vi "Initialize Source Channels.vi"(8 "error in (no error)":errorcluster, 10 "Source Channels":string[](array[string]), 11 "Session in":refnum<k15>) -> (0 "error out":errorcluster, 3 "Session out":refnum<k15>)   [LabVIEW 2020, in "NI-SWITCH Messaging.lvlib" / "NI-SWITCH Consumer.lvclass"]
uses:
  NI-SWITCH Consumer.lvclass
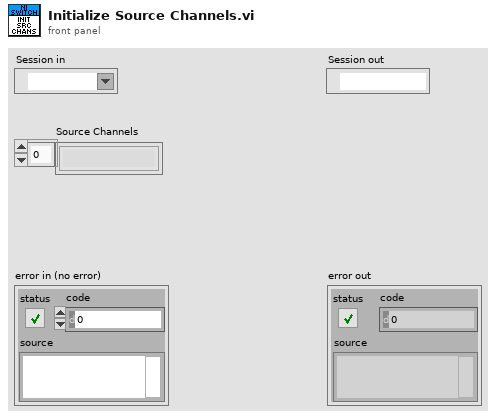
[diagram p1: front panel]
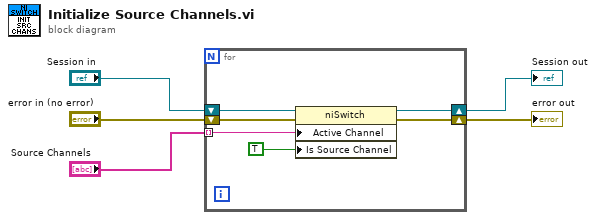
[diagram p0: block diagram]
diagram:
  n1 = for {
    shift-right: [w10] -> w5
    shift-left: "error in (no error)" -> [w11]
    shift-right: [w8] -> w1
    shift-left: "Session in" -> [w9]
    tunnel: "Source Channels" -> [w7] mode=indexing
    n2 = property class="niSwitch"(reference=w9, error in=w11, "Active Channel"=w7, "Is Source Channel"=TRUE ("Channel Configuration:Is Configuration Channel")) -> (reference out=w8:refnum<k15>, error out=w10:errorcluster)
  }
  "error out" <- w5
  "Session out" <- w1
